vi "Read Priority.vi"(8 "error in":errorcluster, 11 "synchronous engine configuration in":refnum<class "synchronous engine configuration.lvclass">) -> (0 "error out":errorcluster, 2 "Priority":i32=1, 3 "synchronous engine configuration out":refnum<class "synchronous engine configuration.lvclass">)   [LabVIEW 2014, in "synchronous engine configuration.lvclass"]
uses:
  synchronous engine configuration.lvclass
  synchronous engine configuration.lvclass/synchronous engine configuration.ctl
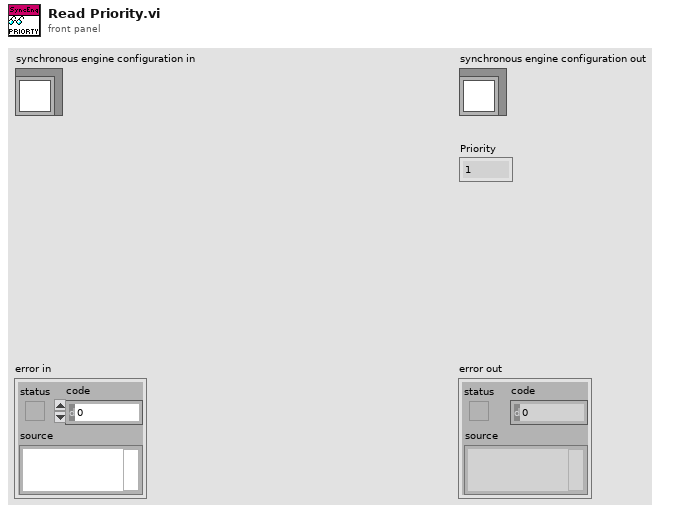
[diagram p1: front panel]
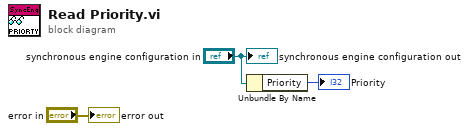
[diagram p0: block diagram]
diagram:
  n1 = Unbundle By Name("synchronous engine configuration in") -> ("Priority"=→"Priority":i32)
  "error out" <- "error in"
  "synchronous engine configuration out" <- "synchronous engine configuration in"
